vi "ESP_tcpTest_server_Multidata.vi"() -> ()   [LabVIEW 2022 SP3]
uses:
  <vilib>/Platform/TimedLoop/XDataNode/timing_clust.ctl
  <vilib>/Platform/TimedLoop/XDataNode/nitl_modes.ctl
  <vilib>/Platform/TimedLoop/XDataNode/wakeup.ctl
  <vilib>/platform/TimedLoop/XDataNode/XDataNode.xnode
  <vilib>/Platform/TimedLoop/XDataNode/XDNodeRunTimeDep.lvlib
panel:
  out "String 2":string
  out "String":string
  out "Potentiometer":dbl(slide) scale=0.0..4095.0
  in  "stop":bool
  out "Potentiometer 2":dbl(slide) scale=0.0..4095.0
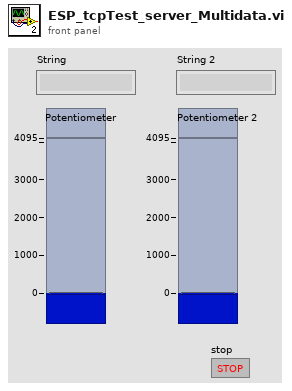
[diagram p1: front panel]
types:
  T1 = typedef "XDNodeRunTimeDep.lvlib/timing_clust.ctl" = cluster{"Expected End [f-1]":u64, "Actual End [f-1]":u64, "Finished Late? [f-1]":bool, "Expected End [i-1]":u64, "Actual End [i-1]":u64, "Finished Late? [i-1]":bool, "Expected Start [i]":u64, "Actual Start [i]":u64, "Expected Start [f]":u64, "Actual Start [f]":u64, "Source Name":string, "Structure Name":string, "Period":i64, "Deadline":i64, "Offset":i64, "Start":i64, "Priority":i32, "Timeout":i32, "Mode":T2, "Wakeup Reason":T3, "Error":errorcluster, "Source Type":string, "Secondary Source Type":string, "Global End Time":u64, "Global Start Time":u64, "Frame Duration":u64, "Iteration Duration":u64, "Assigned CPU":i32, "I/O Scan Engine Mode":u32}
  T2 = typedef "XDNodeRunTimeDep.lvlib/nitl_modes.ctl" = enum32{"No Change", "Process missed periods, maintain original phase", "Discard missed periods, maintain original phase", "Process missed periods, ignore original phase", "Discard missed periods, ignore original phase"}
  T3 = typedef "XDNodeRunTimeDep.lvlib/wakeup.ctl" = enum32{"Normal", "Aborted", "Asynchronous wakeup", "Timing source error", "Timed loop error", "Timeout"}
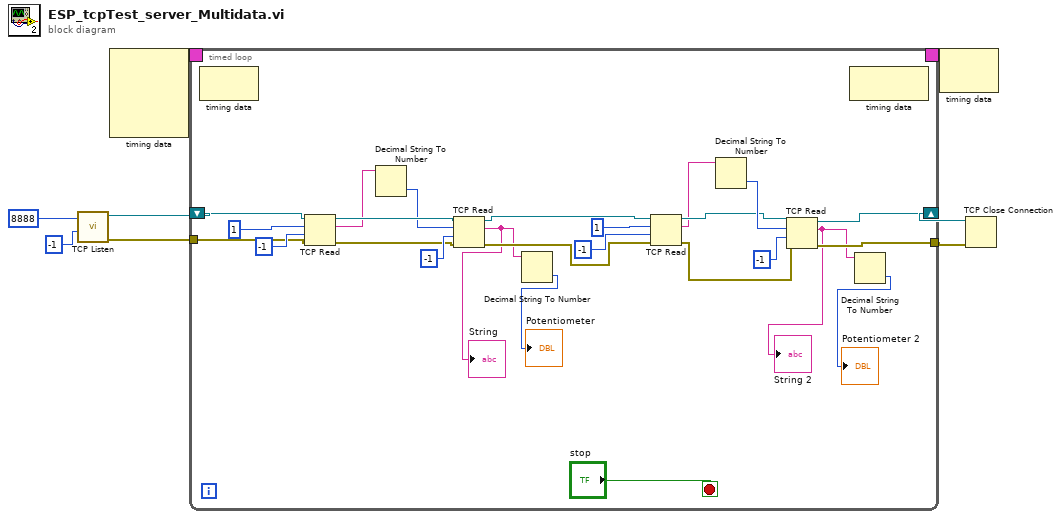
[diagram p0: block diagram]
diagram:
  n1 = call <vilib>:"TCP Listen.vi"("timeout ms (wait forever: -1)"=-1, "port"=u16 8888) -> ("error out"=w3:errorcluster, "connection ID"=w6:refnum<k5>)  [unwired: 5 in, 3 out]
  n2 = node-c288() -> (w8:T1)  [unwired: 4 in]
  n3 = timed-loop {
    timing: w8 -> [_]
    timing-out: [_] -> w7
    shift-right: [w11] -> w1
    shift-left: w6 -> [w33]
    tunnel: w3 -> [w24]
    tunnel: [w19] -> w2
    stop <- "stop" stop-if-true
    n4 = node-c288() -> ()  [unwired: 1 in, 1 out]
    n5 = TCP Read(connection ID=w33, bytes to read=1, error in (no error)=w24, 9:-1 ("timeout ms (25000)")) -> (connection ID out=w29:refnum<k5>, data out=w28:string, error out=w23:errorcluster)  [unwired: 1 in]
    n6 = Decimal String To Number(string=w28) -> (number=w27:i32)  [unwired: 2 in, 1 out]
    n7 = TCP Read(connection ID=w29, bytes to read=w27, error in (no error)=w23, 9:-1 ("timeout ms (25000)")) -> (connection ID out=w17:refnum<k5>, data out=w10:string, error out=w16:errorcluster)  [unwired: 1 in]
    "String" <- w10
    n8 = Decimal String To Number(string=w10) -> (number=→"Potentiometer":i32)  [unwired: 2 in, 1 out]
    n9 = TCP Read(connection ID=w17, bytes to read=1, error in (no error)=w16, 9:-1 ("timeout ms (25000)")) -> (connection ID out=w14:refnum<k5>, data out=w12:string, error out=w13:errorcluster)  [unwired: 1 in]
    n10 = Decimal String To Number(string=w12) -> (number=w20:i32)  [unwired: 2 in, 1 out]
    n11 = TCP Read(connection ID=w14, bytes to read=w20, error in (no error)=w13, 9:-1 ("timeout ms (25000)")) -> (connection ID out=w11:refnum<k5>, data out=w9:string, error out=w19:errorcluster)  [unwired: 1 in]
    "String 2" <- w9
    n12 = node-c288() -> ()  [unwired: 1 in, 1 out]
    n13 = Decimal String To Number(string=w9) -> (number=→"Potentiometer 2":i32)  [unwired: 2 in, 1 out]
  }
  n14 = node-c288(w7) -> ()  [unwired: 1 out]
  n15 = TCP Close Connection(connection ID=w1, error in (no error)=w2) -> ()  [unwired: 1 in, 2 out]
